vi "Viewing JSON Data in a Tree Control.vi"() -> ()   [LabVIEW 2017]
uses:
  <vilib>/National Instruments/Variant Tree Tools/Variant Tree API.lvlib
  <vilib>/National Instruments/Variant JSON API/Variant JSON API.lvlib
panel:
  in  "JSON String":string="[\n  {\n    \"_id\": \"5d411dee05a4243fe140a8b0\",\n    \"index\": 0,\n    \"guid\": \"6649b65f-f9df-468d-a568-878fbbdf55b0\",\n    \"isActive\": false,\n    \"balance\": \"$3,175.92\",\n    \"picture\": \"http://placehold.it/32x32\",\n    \"age\": 21,\n    \"eyeColor\": \"green\",\n    \"name\": \"Deborah Farley\",\n    \"gender\": \"female\",\n    \"company\": \"BULLJUICE\",\n    \"email\": \"deborahfarley@bulljuice.com\",\n    \"phone\": \"+1 (834) 442-2820\",\n    \"address\": \"963 Kensington Walk, Chalfant, Oregon, 5240\",\n    \"about\": \"Quis tempor pariatur consequat sit laborum ipsum magna. Sint nulla excepteur aliquip sunt enim aliquip veniam dolor veniam. Minim eiusmod qui eiusmod aliquip id consequat aute labore minim enim pariatur duis.\\r\\n\",\n    \"registered\": \"2016-02-16T03:44:14 +06:00\",\n    \"latitude\": -64.10574,\n    \"longitude\": -94.872288,\n    \"tags\": [\n      \"sunt\",\n      \"ullamco\",\n      \"anim\",\n      \"incididunt\",\n      \"adipisicing\",\n      \"in\",\n      \"anim\"\n    ],\n    \"friends\": [\n      {\n        \"id\": 0,\n        \"name\": \"Pruitt Vang\"\n      },\n      {\n        \"id\": 1,\n        \"name\": \"Melinda Hayden\"\n      },\n      {\n        \"id\": 2,\n        \"name\": \"Geneva Murphy\"\n      }\n    ],\n    \"greeting\": \"Hello, Deborah Farley! You have 6 unread messages.\",\n    \"favoriteFruit\": \"banana\"\n  },\n  {\n    \"_id\": \"5d411deedde93577e7987f72\",\n    \"index\": 1,\n    \"guid\": \"c06dcd41-b687-4d87-ae5d-535b9b5052b4\",\n    \"isActive\": false,\n    \"balance\": \"$1,735.13\",\n    \"picture\": \"http://placehold.it/32x32\",\n    \"age\": 25,\n    \"eyeColor\": \"blue\",\n    \"name\": \"Maggie Vega\",\n    \"gender\": \"female\",\n    \"company\": \"XELEGYL\",\n    \"email\": \"maggievega@xelegyl.com\",\n    \"phone\": \"+1 (892) 481-2939\",\n    \"address\": \"431 Louisiana Avenue, Lawrence, Maryland, 4856\",\n    \"about\": \"Ullamco aliqua Lorem esse dolor incididunt nisi aliqua. Qui labore incididunt non excepteur eu velit nulla cillum quis enim cupidatat. Labore ea est anim amet incididunt ad id et. Officia nostrud enim sunt cupidatat anim consectetur laboris ad aliqua incididunt mollit do sunt. Minim sit sint consectetur non culpa sunt Lorem dolor ullamco. Irure in aute duis sint nostrud qui culpa ipsum do.\\r\\n\",\n    \"registered\": \"2016-08-02T05:49:42 +05:00\",\n    \"latitude\": -82.77597,\n    \"longitude\": -82.771159,\n    \"tags\": [\n      \"est\",\n      \"labore\",\n      \"nisi\",\n      \"aliqua\",\n      \"labore\",\n      \"voluptate\",\n      \"exercitation\"\n    ],\n    \"friends\": [\n      {\n        \"id\": 0,\n        \"name\": \"Elvia Romero\"\n      },\n      {\n        \"id\": 1,\n        \"name\": \"Lucille Mcpherson\"\n      },\n      {\n        \"id\": 2,\n        \"name\": \"Michelle Baird\"\n      }\n    ],\n    \"greeting\": \"Hello, Maggie Vega! You have 6 unread messages.\",\n    \"favoriteFruit\": \"banana\"\n  },\n  {\n    \"_id\": \"5d411dee60293a9c81ca5ad9\",\n    \"index\": 2,\n    \"guid\": \"f41e7c3d-d5b9-41db-ba10-c105bcd419b1\",\n    \"isActive\": true,\n    \"balance\": \"$2,323.04\",\n    \"picture\": \"http://placehold.it/32x32\",\n    \"age\": 32,\n    \"eyeColor\": \"brown\",\n    \"name\": \"Mae Barron\",\n    \"gender\": \"female\",\n    \"company\": \"QUIZKA\",\n    \"email\": \"maebarron@quizka.com\",\n    \"phone\": \"+1 (933) 593-3832\",\n    \"address\": \"119 Clifton Place, Temperanceville, Puerto Rico, 104\",\n    \"about\": \"Tempor cillum nostrud culpa nulla. Irure velit do ex ex enim ad deserunt consectetur ullamco ullamco adipisicing ut dolor est. Qui veniam et enim elit aliquip exercitation sunt sunt laboris. Pariatur occaecat nulla in ullamco veniam enim reprehenderit duis laborum officia duis deserunt esse nisi.\\r\\n\",\n    \"registered\": \"2018-10-28T09:11:46 +05:00\",\n    \"latitude\": 66.007548,\n    \"longitude\": 155.930841,\n    \"tags\": [\n      \"et\",\n      \"mollit\",\n      \"veniam\",\n      \"do\",\n      \"occaecat\",\n      \"commodo\",\n      \"eiusmod\"\n    ],\n    \"friends\": [\n      {\n        \"id\": 0,\n        \"name\": \"Salas Riggs\"\n      },\n      {\n        \"id\": 1,\n        \"name\": \"Lilly Thomas\"\n      },\n      {\n        \"id\": 2,\n        \"name\": \"Ava Mccoy\"\n      }\n    ],\n    \"greeting\": \"Hello, Mae Barron! You have 7 unread messages.\",\n    \"favoriteFruit\": \"banana\"\n  },\n  {\n    \"_id\": \"5d411deede769e4dd8325c36\",\n    \"index\": 3,\n    \"guid\": \"136cb2b4-7099-4a6c-b6de-1d02703b9eb7\",\n    \"isActive\": false,\n    \"balance\": \"$1,399.61\",\n    \"picture\": \"http://placehold.it/32x32\",\n    \"age\": 22,\n    \"eyeColor\": \"green\",\n    \"name\": \"Peggy Cameron\",\n    \"gender\": \"female\",\n    \"company\": \"EXOTERIC\",\n    \"email\": \"peggycameron@exoteric.com\",\n    \"phone\": \"+1 (858) 486-3139\",\n    \"address\": \"372 Tabor Court, Cuylerville, North Carolina, 1847\",\n    \"about\": \"Deserunt ullamco cupidatat do sunt consequat ex Lorem laborum elit eiusmod. Laboris ullamco eu voluptate commodo occaecat. In occaecat veniam sunt aute dolor ad laborum sit occaecat consequat ut non proident. Ad pariatur ad ullamco mollit commodo elit ex duis anim Lorem pariatur laborum enim reprehenderit. Deserunt exercitation non esse labore minim aute.\\r\\n\",\n    \"registered\": \"2014-04-02T07:07:27 +05:00\",\n    \"latitude\": -53.506506,\n    \"longitude\": 29.433646,\n    \"tags\": [\n      \"consequat\",\n      \"et\",\n      \"ipsum\",\n      \"ipsum\",\n      \"duis\",\n      \"cupidatat\",\n      \"magna\"\n    ],\n    \"friends\": [\n      {\n        \"id\": 0,\n        \"name\": \"Marianne Callahan\"\n      },\n      {\n        \"id\": 1,\n        \"name\": \"Beatrice Wheeler\"\n      },\n      {\n        \"id\": 2,\n        \"name\": \"Shields Vance\"\n      }\n    ],\n    \"greeting\": \"Hello, Peggy Cameron! You have 8 unread messages.\",\n    \"favoriteFruit\": \"banana\"\n  },\n  {\n    \"_id\": \"5d411dee2f63c611bf50e15b\",\n    \"index\": 4,\n    \"guid\": \"6bf3b75d-2921-4175-a12f-363f2b838c45\",\n    \"isActive\": false,\n    \"balance\": \"$1,022.91\",\n    \"picture\": \"http://placehold.it/32x32\",\n    \"age\": 35,\n    \"eyeColor\": \"green\",\n    \"name\": \"Ford Payne\",\n    \"gender\": \"male\",\n    \"company\": \"IMANT\",\n    \"email\": \"fordpayne@imant.com\",\n    \"phone\": \"+1 (917) 407-2977\",\n    \"address\": \"376 Manhattan Court, Irwin, Alabama, 4516\",\n    \"about\": \"Quis exercitation exercitation non excepteur culpa aute minim eiusmod mollit eu ex in id cillum. Sint culpa et sint minim dolor est est aliqua culpa non occaecat. In quis duis dolore ut do nostrud voluptate est nisi cillum.\\r\\n\",\n    \"registered\": \"2014-12-07T01:52:08 +06:00\",\n    \"latitude\": -75.34591,\n    \"longitude\": 135.968465,\n    \"tags\": [\n      \"ipsum\",\n      \"officia\",\n      \"exercitation\",\n      \"laborum\",\n      \"Lorem\",\n      \"deserunt\",\n      \"et\"\n    ],\n    \"friends\": [\n      {\n        \"id\": 0,\n        \"name\": \"Marla Hatfield\"\n      },\n      {\n        \"id\": 1,\n        \"name\": \"Green Burris\"\n      },\n      {\n        \"id\": 2,\n        \"name\": \"Davenport Glenn\"\n      }\n    ],\n    \"greeting\": \"Hello, Ford Payne! You have 6 unread messages.\",\n    \"favoriteFruit\": \"apple\"\n  },\n  {\n    \"_id\": \"5d411dee610494d2f5ccb62c\",\n    \"index\": 5,\n    \"guid\": \"36d8a9d4-d1f4-46f4-941e-99b429a5e1cf\",\n    \"isActive\": false,\n    \"balance\": \"$3,754.36\",\n    \"picture\": \"http://placehold.it/32x32\",\n    \"age\": 24,\n    \"eyeColor\": \"blue\",\n    \"name\": \"Garrison Richmond\",\n    \"gender\": \"male\",\n    \"company\": \"EGYPTO\",\n    \"email\": \"garrisonrichmond@egypto.com\",\n    \"phone\": \"+1 (981) 524-2642\",\n    \"address\": \"902 Atlantic Avenue, Crawfordsville, Illinois, 7709\",\n    \"about\": \"Velit adipisicing sunt exercitation ut adipisicing veniam ad nostrud aliquip ipsum enim. Ad pariatur sint dolor mollit aliqua nulla qui et eu consectetur velit do ad. Aliqua ex culpa eiusmod excepteur laborum dolore. Ipsum minim anim voluptate aliquip nostrud enim. Duis velit ipsum pariatur amet qui incididunt qui sit aliquip nulla.\\r\\n\",\n    \"registered\": \"2016-08-02T04:16:22 +05:00\",\n    \"latitude\": 51.85107,\n    \"longitude\": -162.856836,\n    \"tags\": [\n      \"aute\",\n      \"ut\",\n      \"nisi\",\n      \"consequat\",\n      \"fugiat\",\n      \"labore\",\n      \"aliqua\"\n    ],\n    \"friends\": [\n      {\n        \"id\": 0,\n        \"name\": \"Mollie Carey\"\n      },\n      {\n        \"id\": 1,\n        \"name\": \"Theresa Horton\"\n      },\n      {\n        \"id\": 2,\n        \"name\": \"Brenda Horn\"\n      }\n    ],\n    \"greeting\": \"Hello, Garrison Richmond! You have 8 unread messages.\",\n    \"favoriteFruit\": \"banana\"\n  },\n  {\n    \"_id\": \"5d411dee3c51bb611a4ac51d\",\n    \"index\": 6,\n    \"guid\": \"bb9254f2-3f15-4456-90c5-e6929552a0e8\",\n    \"isActive\": true,\n    \"balance\": \"$1,960.79\",\n    \"picture\": \"http://placehold.it/32x32\",\n    \"age\": 21,\n    \"eyeColor\": \"brown\",\n    \"name\": \"Elnora Hughes\",\n    \"gender\": \"female\",\n    \"company\": \"COMBOGEN\",\n    \"email\": \"elnorahughes@combogen.com\",\n    \"phone\": \"+1 (876) 413-3289\",\n    \"address\": \"173 Billings Place, Bannock, South Dakota, 6298\",\n    \"about\": \"Sunt qui aute irure exercitation laboris aute Lorem adipisicing et consectetur consequat adipisicing quis dolor. Aliqua elit esse sit et ipsum est ex culpa laboris do ipsum. Magna magna magna cupidatat tempor minim dolore sunt irure. Qui culpa aute do incididunt. Fugiat veniam ut laboris enim Lorem magna enim do non minim. Amet commodo dolor pariatur esse cillum deserunt commodo in excepteur reprehenderit.\\r\\n\",\n    \"registered\": \"2015-09-24T04:54:33 +05:00\",\n    \"latitude\": -85.736049,\n    \"longitude\": -125.914804,\n    \"tags\": [\n      \"excepteur\",\n      \"consectetur\",\n      \"adipisicing\",\n      \"excepteur\",\n      \"qui\",\n      \"labore\",\n      \"duis\"\n    ],\n    \"friends\": [\n      {\n        \"id\": 0,\n        \"name\": \"English Pena\"\n      },\n      {\n        \"id\": 1,\n        \"name\": \"Sheena Lee\"\n      },\n      {\n        \"id\": 2,\n        \"name\": \"Skinner Grimes\"\n      }\n    ],\n    \"greeting\": \"Hello, Elnora Hughes! You have 5 unread messages.\",\n    \"favoriteFruit\": \"apple\"\n  }\n]"
  in  "Tree":string(tree)
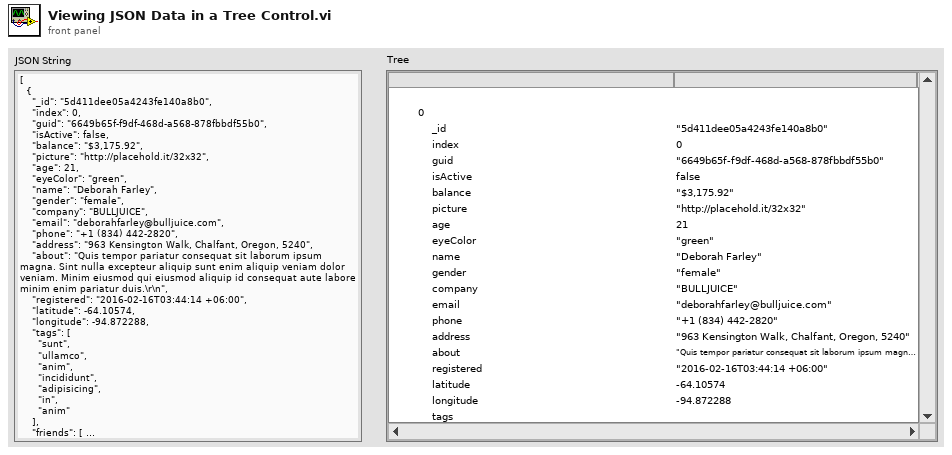
[diagram p1: front panel]
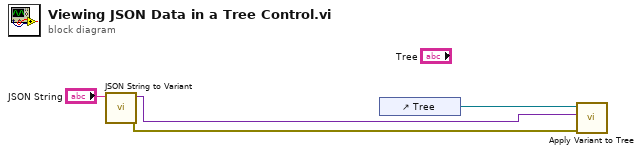
[diagram p0: block diagram]
diagram:
  n1 = call <vilib>:"JSON String to Variant.vi"("JSON String"="JSON String") -> ("error out"=w1:errorcluster, "Variant out"=w3:variant)  [unwired: 9 in]
  n2 = control-ref of="Tree"() -> (w4:refnum<vi>)
  n3 = call <vilib>:"Apply Variant to Tree.vi"("error in (no error)"=w1, "Variant"=w3, "TreeControl in"=w4) -> ()  [unwired: 7 in, 2 out]
